vi "Message.vi"(8 "error in (no error)":errorcluster) -> (0 "error out":errorcluster)   [LabVIEW 2023]
uses:
  Log.lvclass
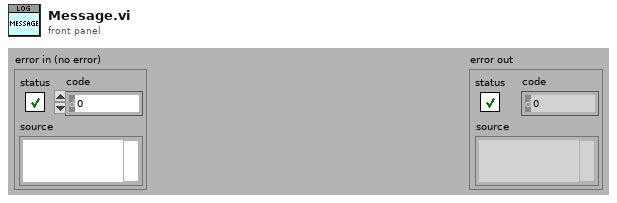
[diagram p1: front panel]
types:
  T1 = typedef "Log.lvclass/ObjectAttributes.ctl" = cluster{"Level":T2, "Facilities":variant, "Event":refnum<user-event>}
  T2 = typedef "Log.lvclass/Log_Level.ctl" = enum16{"none", "info", "trace", "warn", "error", "fatal"}
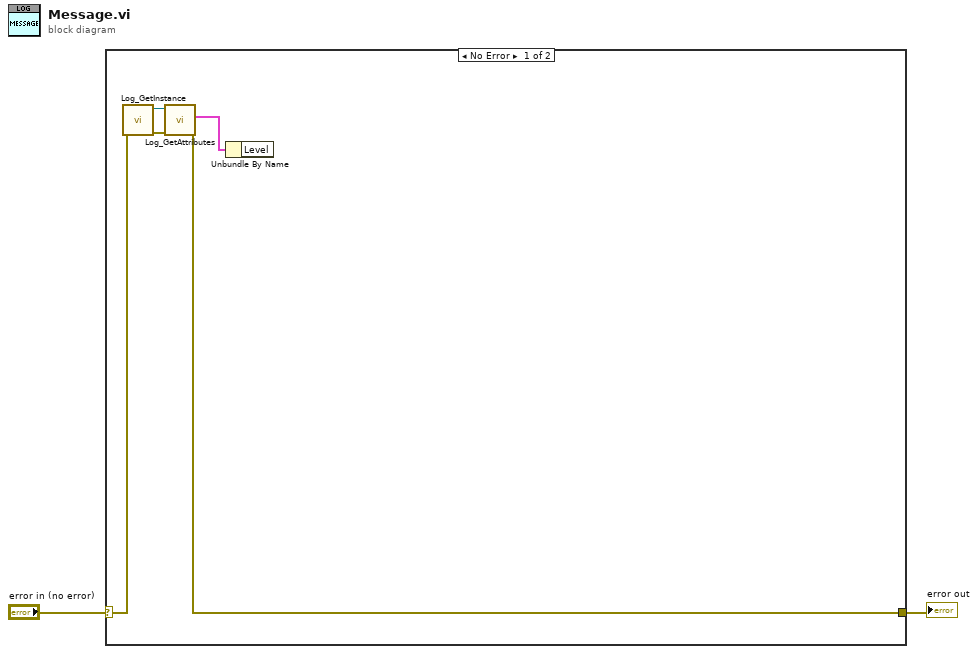
[diagram p0: block diagram]
diagram:
  n1 = case shown="No Error" "error in (no error)" {
    selector: "error in (no error)" -> [w4 w8]
    tunnel: [w6 w8] -> w1
    frame No Error {
      n2 = call "Log_GetInstance.vi"("error in (no error)"=w4) -> ("error out"=w3:errorcluster, "reference out"=w5:refnum<class "Log.lvclass">)  [unwired: 6 in, 3 out]
      n3 = call "Log_GetAttributes.vi"("error in (no error)"=w3, "reference in"=w5) -> ("error out"=w6:errorcluster, "Data"=w7:T1)  [unwired: 6 in, 2 out]
      n4 = Unbundle By Name(w7) -> ()  [unwired: 1 out]
    }
    frame Error {
    }
  }
  "error out" <- w1
